vi "Test-TimeToString.vi"() -> ()   [LabVIEW 2014]
panel:
  out "当前时间":timestamp
  out "*(类型 *) &x 2":timestamp
  out "大小 3":i32
  out "大小 2":i32
  out "字符串":string
  out "*(类型 *) &x":string
  out "大小":i32
  out "日期/时间字符串":string
  in  "起始时间":timestamp=timestamp(3515993400.420156 s since 1904-01-01)
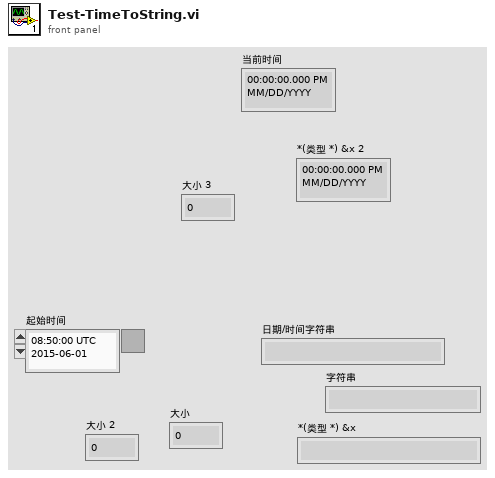
[diagram p1: front panel]
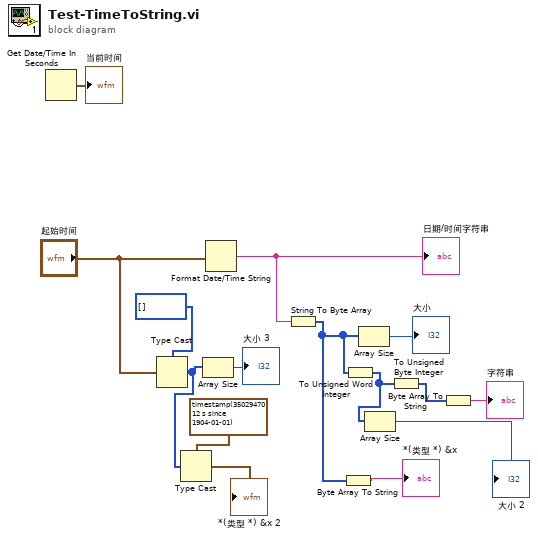
[diagram p0: block diagram]
diagram:
  n1 = Get Date/Time In Seconds() -> (seconds since 1Jan1904=→"当前时间":timestamp)
  n2 = Type Cast(type=u16[] [], x="起始时间") -> (*(type *) &x=w4:u16[])
  n3 = Type Cast(type=timestamp(3502947012.42 s since 1904-01-01) ("起始时间"), x=w4) -> (*(type *) &x=→"*(类型 *) &x 2":timestamp)
  n4 = Array Size(array=w4) -> (size(s)=→"大小 3":i32)
  n5 = Format Date/Time String(seconds (now)="起始时间") -> (date/time string=w14:string)  [unwired: 2 in]
  "日期/时间字符串" <- w14
  n6 = String To Byte Array(string=w14) -> (unsigned byte array=w12:u8[])
  n7 = Byte Array To String(unsigned byte array=w12) -> (string=→"*(类型 *) &x":string)
  n8 = To Unsigned Word Integer(number=w12) -> (unsigned 16bit integer=w9:u16[])
  n9 = Array Size(array=w12) -> (size(s)=→"大小":i32)
  n10 = Array Size(array=w9) -> (size(s)=→"大小 2":i32)
  n11 = To Unsigned Byte Integer(number=w9) -> (unsigned 8bit integer=w11:u8[])
  n12 = Byte Array To String(unsigned byte array=w11) -> (string=→"字符串":string)
